vi "Counter.vi"() -> (3 "数值":u32)   [LabVIEW 2015, in "Timed Loop Actor.lvlib" / "Timed Loop Actor.lvclass"]
uses:
  Timed Loop Actor.lvclass
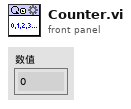
[diagram p1: front panel]
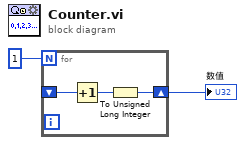
[diagram p0: block diagram]
diagram:
  n1 = for {
    N: 1 -> [_]
    shift-right: [w4] -> w2
    shift-left: _ -> [w3]
    n2 = Increment(x=w3) -> (x+1=w5:u32)
    n3 = To Unsigned Long Integer(number=w5) -> (unsigned 32bit integer=w4:u32)
  }
  "数值" <- w2
